vi "sub_create tasks.vi"(1 "DAQ Sample Rate":dbl) -> (0 "output cluster":T1)   [LabVIEW 2021]
uses:
  <vilib>/ULx/ULx_LV.dll
  <vilib>/DAQmx/create/channels.llb/DAQmx Create Channel (AO-Voltage-Basic).vi
  <vilib>/DAQmx/configure/timing.llb/DAQmx Timing (Sample Clock).vi
  globalvariables.vi
  <vilib>/DAQmx/create/channels.llb/DAQmx Create Channel (AI-Voltage-Basic).vi
  <vilib>/ULx/Timing.llb/ULx Timing (Sample Clock).vi
  <resource>/objmgr/daqmx.rc
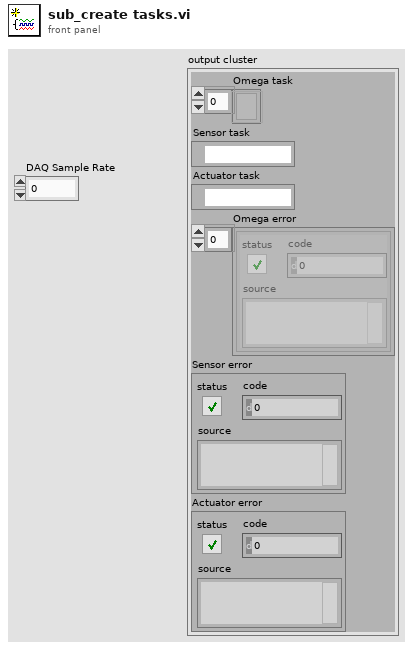
[diagram p1: front panel]
types:
  T1 = cluster{"Omega task":refnum<k24>[], "Sensor task":refnum<k21>, "Actuator task":refnum<k21>, "Omega error":errorcluster[], "Sensor error":errorcluster, "Actuator error":errorcluster}
  T2 = cluster{refnum<k24>[], "task out":refnum<k21>, "task out":refnum<k21>, errorcluster[], "error out":errorcluster, "error out":errorcluster}
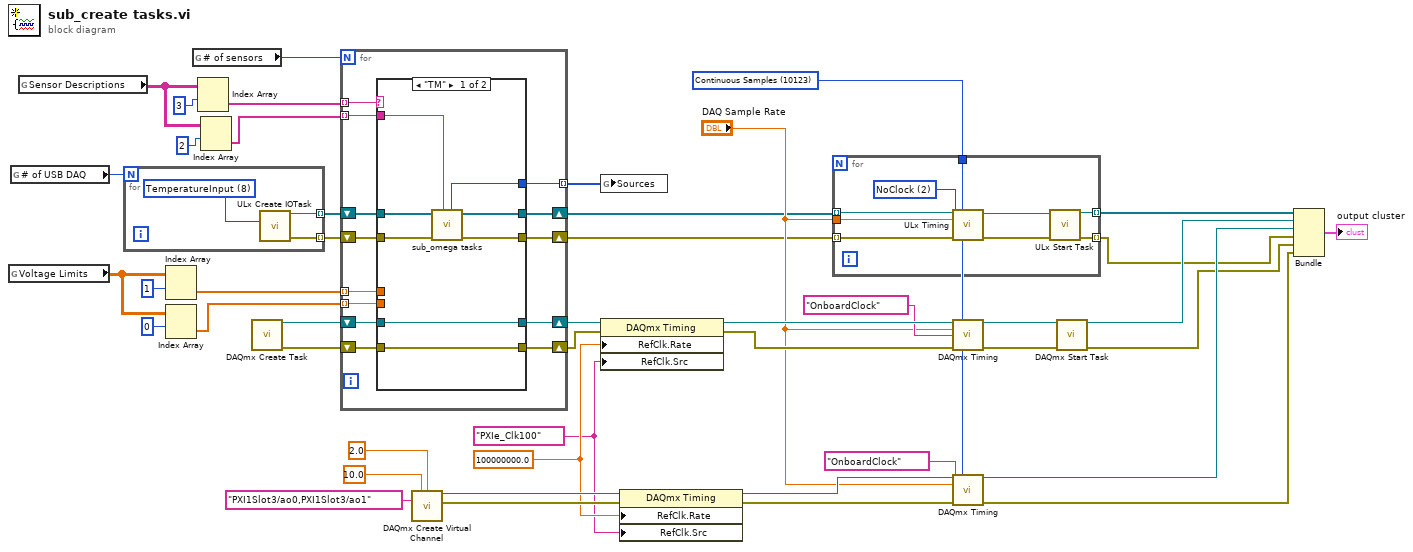
[diagram p0: block diagram]
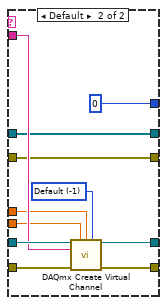
[diagram p2: hidden frame]
diagram:
  w21 = 100000000.0 ("SampClk.Rate")
  w20 = tag "PXIe_Clk100" ("SampClk.Src")
  w15 = 10123 items=["Finite Samples"=10178, "Continuous Samples"=10123, "Hardware Timed Single Point"=12522] ("sample mode")
  n1 = global read "globalvariables.vi" "Voltage Limits"() -> (w18:dbl[][])
  n2 = global read "globalvariables.vi" "# of USB DAQ"() -> (w12:i32)
  n3 = global read "globalvariables.vi" "Sensor Descriptions"() -> (w19:string[][])
  n4 = for {
    N: w12 -> [_]
    tunnel: [w48] -> w14 mode=indexing
    tunnel: [w47] -> w13 mode=indexing
    w46 = 8 items=["AnalogInput", "AnalogOutput", "DigitalInput", "DigitalOutput", "CounterInput", "CounterOutput", "CompositeInput", "CompositeOutput", "TemperatureInput"] ("taskType")
    n5 = call <vilib>:"ULx Create IOTask.vi"("taskType"=w46) -> ("error out"=w47:errorcluster, "i/o task out"=w48:refnum<k24>)  [unwired: 9 in]
  }
  n6 = Index Array(array=w18, index (row)=1) -> (element=w25:dbl[])  [unwired: 1 in]
  n7 = Index Array(array=w18, index (row)=0) -> (element=w24:dbl[])  [unwired: 1 in]
  n8 = global read "globalvariables.vi" "# of sensors"() -> (w17:i32)
  n9 = Index Array(array=w19, index (row)=3) -> (element=w23:string[])  [unwired: 1 in]
  n10 = Index Array(array=w19, index (row)=2) -> (element=w22:string[])  [unwired: 1 in]
  n11 = call <vilib>:"DAQmx Create Task.vi"() -> ("task out"=w30:refnum<k21>, "error out"=w29:errorcluster)  [unwired: 14 in]
  n12 = for {
    N: w17 -> [_]
    tunnel: w22 -> [w57] mode=indexing
    shift-right: [w59] -> w26
    shift-left: w29 -> [w61]
    shift-right: [w58] -> w27
    shift-left: w30 -> [w60]
    tunnel: w25 -> [w56] mode=indexing
    tunnel: w24 -> [w55] mode=indexing
    tunnel: w23 -> [w54] mode=indexing
    tunnel: [w53] -> w9 mode=indexing
    shift-right: [w49] -> w11
    shift-left: w13 -> [w51]
    shift-right: [w50] -> w10
    shift-left: w14 -> [w52]
    n13 = case shown="\"TM\"" w54 {
      tunnel: w61 -> [w69 w80]
      tunnel: w60 -> [w68 w79]
      tunnel: [w69 w78] -> w59
      tunnel: [w68 w77] -> w58
      tunnel: w57 -> [w64 w75]
      tunnel: w56 -> [_ w74]
      tunnel: w55 -> [_ w73]
      tunnel: [w67 0] -> w53
      tunnel: w52 -> [w63 w72]
      tunnel: w51 -> [w65 w71]
      tunnel: [w62 w72] -> w50
      tunnel: [w66 w71] -> w49
      frame "TM" {
        n14 = call "sub_omega tasks.vi"("DAQ Channel"=w64, "Omega errors"=w65, "Omega tasks"=w63) -> ("Omega errors out"=w66:errorcluster[], "Omega tasks out"=w62:refnum<k24>[], "Source Number"=w67:i32)  [unwired: 4 in]
      }
      frame Default {
        w76 = -1 items=["Default"=-1, "RSE"=10083, "NRSE"=10078, "Differential"=10106, "Pseudodifferential"=12529] ("input terminal configuration")
        n15 = call-poly <vilib>:"DAQmx Create Virtual Channel.vi"("task in"=w79, "maximum value"=w73, "minimum value"=w74, "input terminal configuration"=w76, "physical channels"=w75, "error in"=w80) -> ("task out"=w77:refnum<k21>, "error out"=w78:errorcluster)  [unwired: 8 in]
      }
    }
  }
  n16 = call-poly <vilib>:"DAQmx Create Virtual Channel.vi"("maximum value"=10.0, "minimum value"=2.0, "physical channels"=tag "PXI1Slot3/ao0,PXI1Slot3/ao1") -> ("task out"=w39:refnum<k21>, "error out"=w40:errorcluster)  [unwired: 11 in]
  n17 = global write "globalvariables.vi" "Sources"(w9) -> ()
  n18 = property class="DAQmx Timing"(reference=w27, error in=w26, "RefClk.Rate"=w21, "RefClk.Src"=w20) -> (reference out=w33:refnum<k21>, error out=w34:errorcluster)
  n19 = property class="DAQmx Timing"(reference=w39, error in=w40, "RefClk.Rate"=w21, "RefClk.Src"=w20) -> (reference out=w41:refnum<k21>, error out=w42:errorcluster)
  n20 = for {
    tunnel: w10 -> [w85] mode=indexing
    tunnel: w11 -> [w86] mode=indexing
    tunnel: [w82] -> w8 mode=indexing
    tunnel: [w81] -> w4 mode=indexing
    tunnel: w15 -> [w88]
    tunnel: "DAQ Sample Rate" -> [w89]
    w87 = 2 items=["OnboardClock", "ExternalClock", "NoClock"] ("clock source")
    n21 = call-poly <vilib>:"ULx Timing.vi"("task in"=w85, "sample mode"=w88, "rate"=w89, "clock source"=w87, "error in"=w86) -> ("task out"=w84:refnum<k24>, "error out"=w83:errorcluster)  [unwired: 9 in]
    n22 = call <vilib>:"ULx Start Task.vi"("task in"=w84, "error in"=w83) -> ("task out"=w82:refnum<k24>, "error out"=w81:errorcluster)  [unwired: 12 in]
  }
  n23 = call-poly <vilib>:"DAQmx Timing.vi"("task/channels in"=w33, "sample mode"=w15, "rate"="DAQ Sample Rate", "source"=tag "OnboardClock", "error in"=w34) -> ("task out"=w32:refnum<k21>, "error out"=w31:errorcluster)  [unwired: 9 in]
  n24 = call-poly <vilib>:"DAQmx Timing.vi"("task/channels in"=w41, "sample mode"=w15, "rate"="DAQ Sample Rate", "source"=tag "OnboardClock", "error in"=w42) -> ("task out"=w5:refnum<k21>, "error out"=w2:errorcluster)  [unwired: 9 in]
  n25 = call <vilib>:"DAQmx Start Task.vi"("task/channels in"=w32, "error in"=w31) -> ("task out"=w7:refnum<k21>, "error out"=w3:errorcluster)  [unwired: 12 in]
  n26 = Bundle(w8, "task out"=w7, "task out"=w5, w4, "error out"=w3, "error out"=w2) -> (→"output cluster":T2)  [unwired: 1 in]
